vi "Kinematyka prosta.vi"(5 "Parametry robota":T2={"Promień koła [m]"=0.045, "Szerokość robota [m]"=0.37}, 6 "Początkowa odległość robota od startu":T1, 7 "Orientacja pocz. [stopnie]":dbl, 8 "Orientacja [stopnie]":dbl, 9 "Prędkość kątowa prawych kół [rad/s]":dbl, 10 "Prędkość kątowa lewych kół [rad/s]":dbl) -> (1 "Orientacja kąt [stopnie]":dbl format="%.9f", 2 "Odległość robota od startu":cluster{"X[m]":dbl, "Y[m]":dbl} {"Y[m]" format="%.9f"; "X[m]" format="%.9f"})   [LabVIEW 2012]
doc: "Plik odpowiedzialny za wyznaczenie kinematyki prostej badanego robota (typu skid-steering z uproszczeniem do kinematyki typu differenttial drive). Jako zmienne wejściowe podawane są prędkości kątowe z enkoderów odpowiednio przeskalowane do jednostek czasu.\nNa wyjściu otrzymujemy położenie robota i kąt pod jakim się znajduje w stosunku do układu bazowego."
panel:
  # "Odległość robota od położenia początkowego w zależności \nod prędkości kątowej kół i orientacji robota"
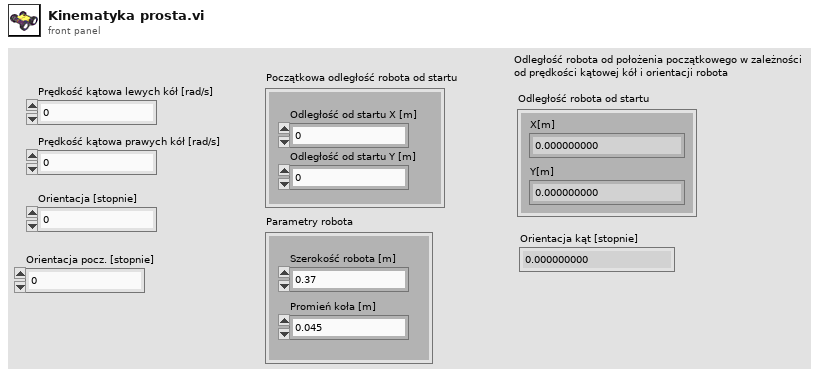
[diagram p1: front panel]
types:
  T1 = cluster{"Odległość od startu X [m]":dbl, "Odległość od startu Y [m]":dbl}
  T2 = cluster{"Promień koła [m]":dbl, "Szerokość robota [m]":dbl}
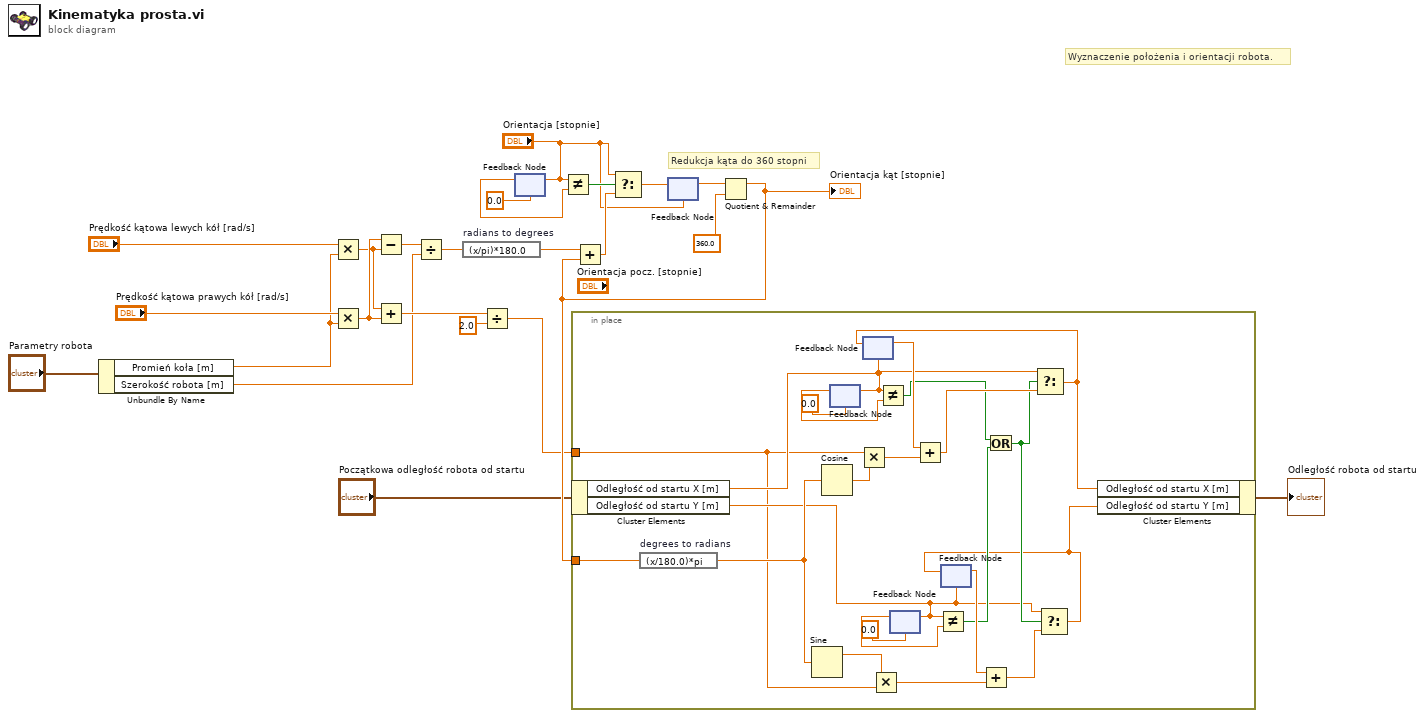
[diagram p0: block diagram]
diagram:
  # "Wyznaczenie położenia i orientacji robota."
  # "Redukcja kąta do 360 stopni"
  n1 = Unbundle By Name("Parametry robota") -> ("Promień koła [m]"=w11:dbl, "Szerokość robota [m]"=w10:dbl)
  n2 = Multiply(x="Prędkość kątowa lewych kół [rad/s]", y=w11) -> (x*y=w20:dbl)
  n3 = Multiply(x="Prędkość kątowa prawych kół [rad/s]", y=w11) -> (x*y=w21:dbl)
  n4 = Subtract(x=w21, y=w20) -> (x-y=w19:dbl)
  n5 = Add(x=w20, y=w21) -> (x+y=w23:dbl)
  n6 = Divide(x=w19, y=w10) -> (x/y=w18:dbl)
  n7 = expression code="(x/pi)*180.0" "radians to degrees"(w18) -> (w17:dbl)
  n8 = Divide(x=w23, y=2.0) -> (x/y=w5:dbl)
  n9 = feedback #1(0.0 ("Y")) -> (w8:dbl)
  n10 = feedback-in #1("Orientacja [stopnie]") -> ()
  n11 = Not Equal?(x="Orientacja [stopnie]", y=w8) -> (x != y?=w7:bool)
  n12 = feedback #2("Orientacja [stopnie]") -> (w2:dbl)
  n13 = Quotient & Remainder(x=w2, y=360.0) -> (x-y*floor(x/y)=w13:dbl)  [unwired: 1 out]
  "Orientacja kąt [stopnie]" <- w13
  n14 = in-place {
    in-place-border: w5 -> [w25]
    in-place-border: w13 -> [w37]
    n15 = in-place-cluster #3("Początkowa odległość robota od startu") -> ("Odległość od startu X [m]"=w29:dbl, "Odległość od startu Y [m]"=w28:dbl)
    n16 = expression code="(x/180.0)*pi" "degrees to radians"(w37) -> (w45:dbl)
    n17 = Sine(x=w45) -> (sin(x)=w38:dbl)
    n18 = Cosine(x=w45) -> (cos(x)=w46:dbl)
    n19 = feedback #4(0.0 ("Y")) -> (w33:dbl)
    n20 = feedback-in #4(w29) -> ()
    n21 = Multiply(x=w25, y=w46) -> (x*y=w41:dbl)
    n22 = feedback #5(w29) -> (w42:dbl)
    n23 = Multiply(x=w38, y=w25) -> (x*y=w39:dbl)
    n24 = Not Equal?(x=w29, y=w33) -> (x != y?=w32:bool)
    n25 = feedback #6(0.0 ("Y")) -> (w35:dbl)
    n26 = feedback-in #6(w28) -> ()
    n27 = Add(x=w42, y=w41) -> (x+y=w44:dbl)
    n28 = Not Equal?(x=w28, y=w35) -> (x != y?=w31:bool)
    n29 = feedback #7(w28) -> (w40:dbl)
    n30 = Add(x=w40, y=w39) -> (x+y=w43:dbl)
    n31 = Or(x=w32, y=w31) -> (x .or. y?=w30:bool)
    n32 = Select(t=w29, s=w30, f=w44) -> (s? t:f=w27:dbl)
    n33 = feedback-in #5(w27) -> ()
    n34 = Select(t=w28, s=w30, f=w43) -> (s? t:f=w26:dbl)
    n35 = feedback-in #7(w26) -> ()
    n36 = in-place-cluster #3("Odległość od startu X [m]"=w27, "Odległość od startu Y [m]"=w26) -> (→"Odległość robota od startu":T1)
  }
  n37 = Add(x=w17, y=w13) -> (x+y=w15:dbl)
  n38 = Select(t="Orientacja [stopnie]", s=w7, f=w15) -> (s? t:f=w3:dbl)
  n39 = feedback-in #2(w3) -> ()
